vi "projet_licence_1.vi"() -> ()   [LabVIEW 2021]
uses:
  <vilib>/addons/control/pid/pid.llb/PID (DBL).vi
  <vilib>/addons/control/pid/NI_PID_pid.lvlib
panel:
  in  "Température\nde consigne":dbl=20.0 min=20.0 max=50.0 format="%#_4g"
  out "PWM correspondant":u8
  in  "Pin":u8=1 caption="Pin [0 - 11]" max=11
  out "Waveform Chart 2":dynamicdata(graph)
  in  "Commande onglet":T1(tab)
  out "Température mesurée":dbl
  out "Température mesurée":dbl(slide) scale=0.0..100.0
  out "Température actuelle":dbl
  out "Température mesurée":dbl(slide) scale=0.0..100.0
  in  "Température\nde consigne":dbl=20.0 min=20.0 max=50.0 format="%#_4g"
  out "Tension de consigne correspondante":dbl
  out "Température mesurée":dbl(slide) scale=0.0..100.0
  in  "Température de consigne":dbl(slide) scale=0.0..100.0
  out "Erreur":dbl
  out "Température":dbl(slide) scale=0.0..100.0
  out "Température actuelle":dbl
  in  "PID gains":T2={"derivative time (Td, min)"=0.0, "integral time (Ti, min)"=0.01, "proportional gain (Kc)"=1.0} {"proportional gain (Kc)" format="%.3f"; "integral time (Ti, min)" format="%.3f"; "derivative time (Td, min)" format="%.3f"}
  in  "stop":bool
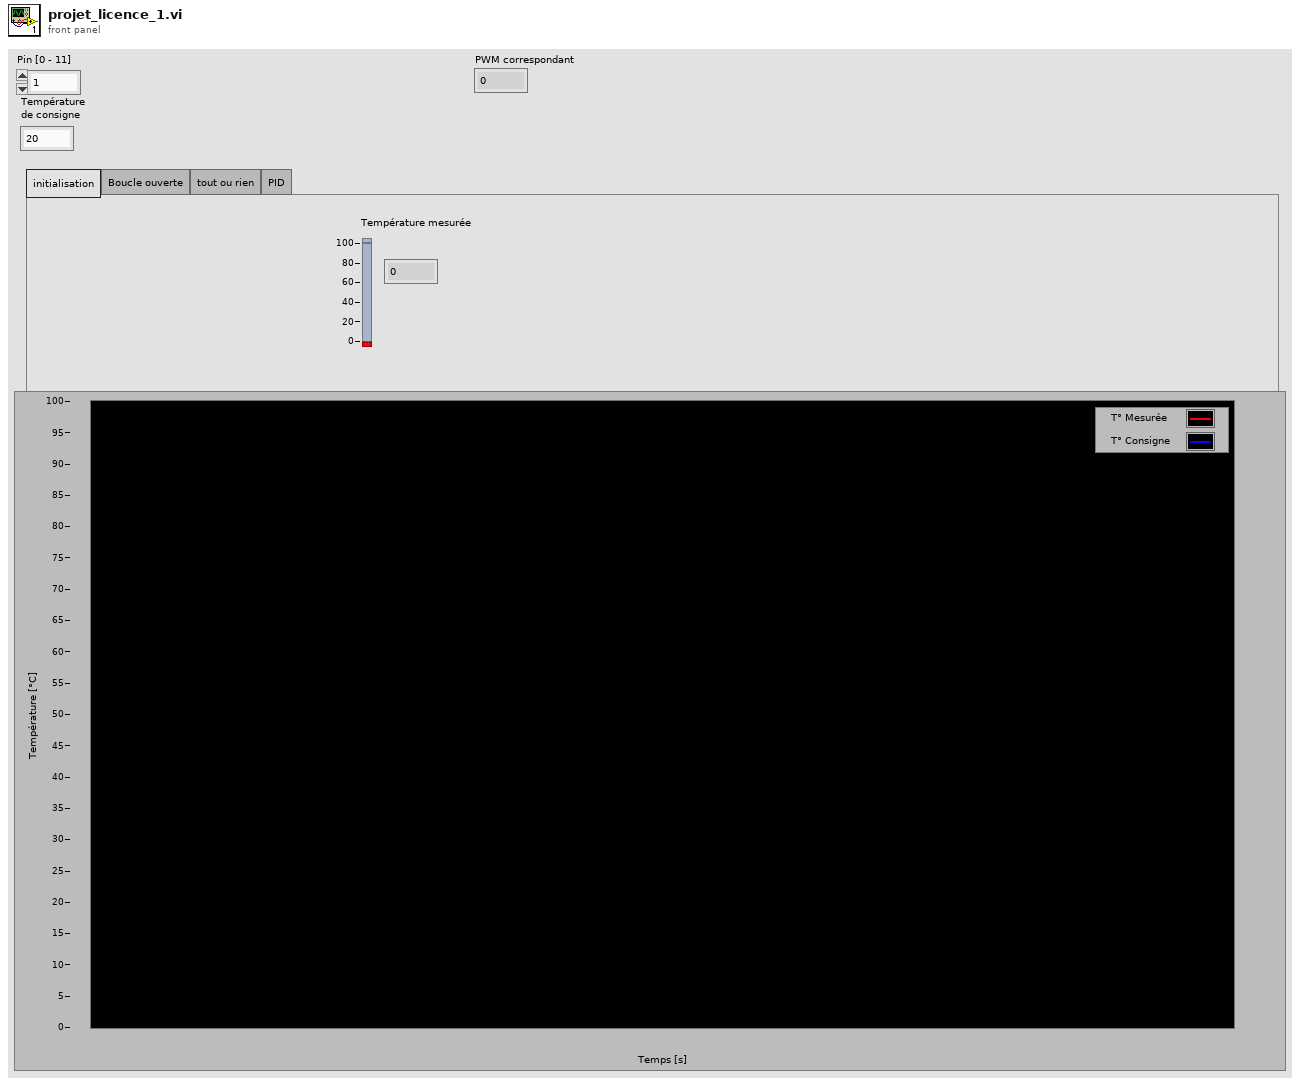
[diagram p1: front panel]
types:
  T1 = enum32{"initialisation", "Boucle ouverte", "tout ou rien", "PID"}
  T2 = cluster{"derivative time (Td, min)":dbl, "integral time (Ti, min)":dbl, "proportional gain (Kc)":dbl}
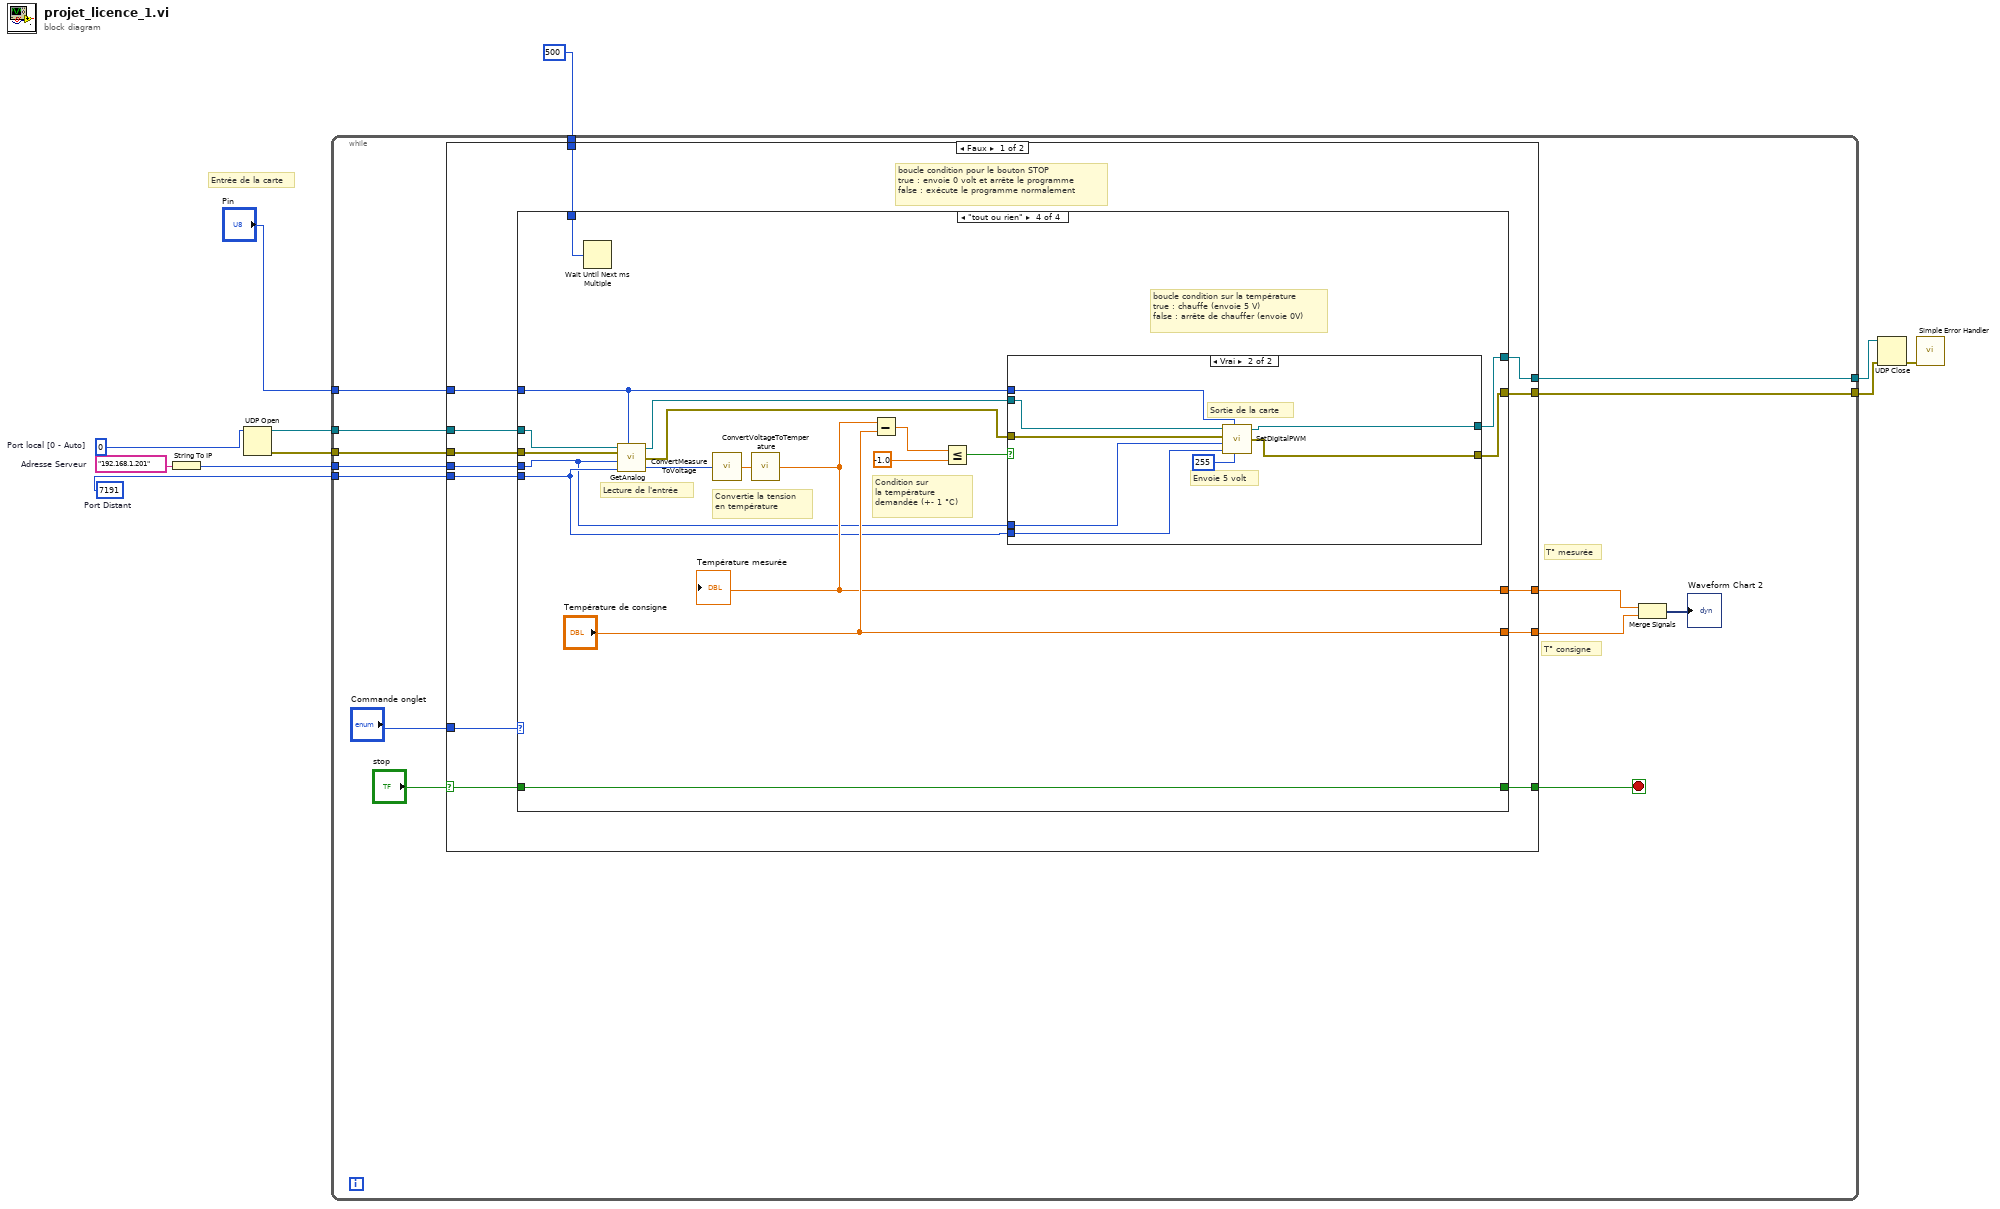
[diagram p0: block diagram]
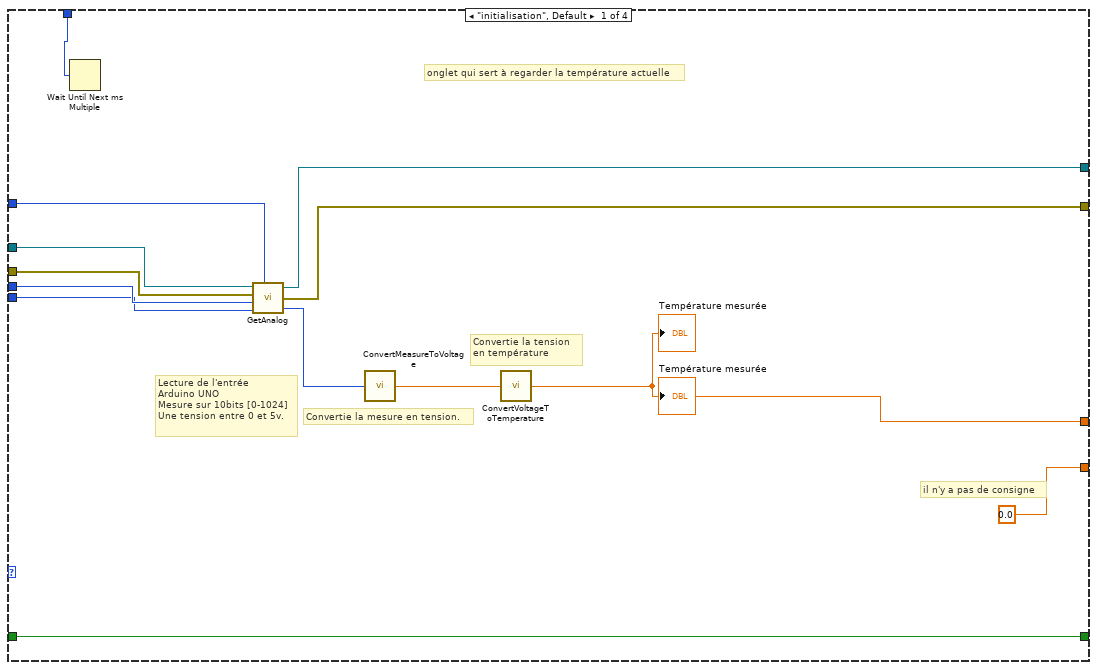
[diagram p2: hidden frame]
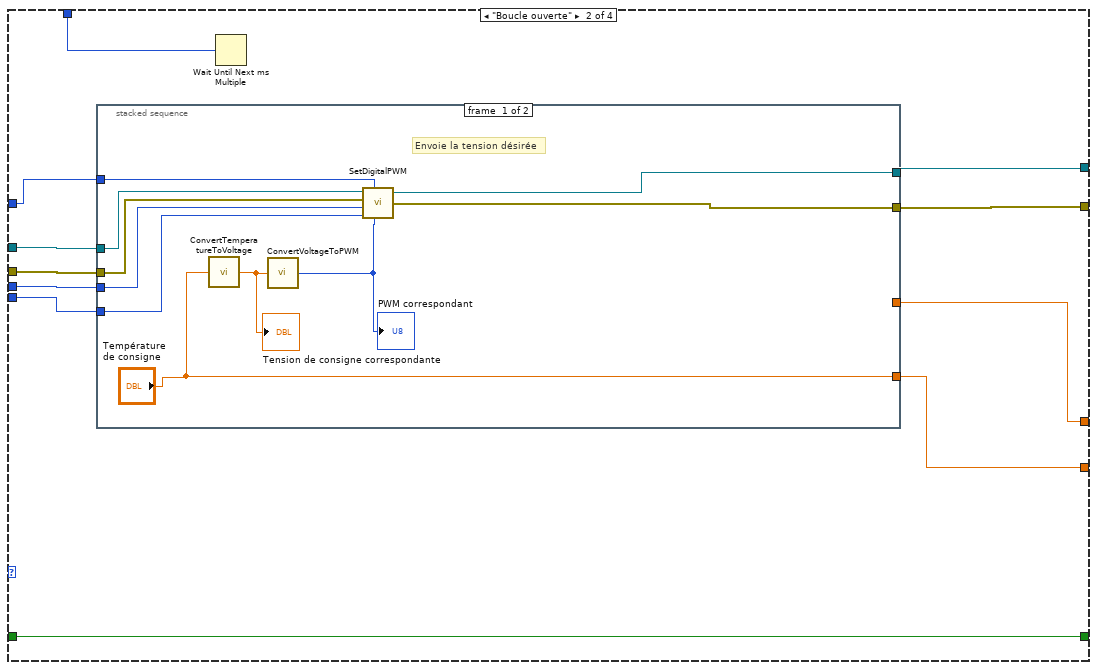
[diagram p3: hidden frame]
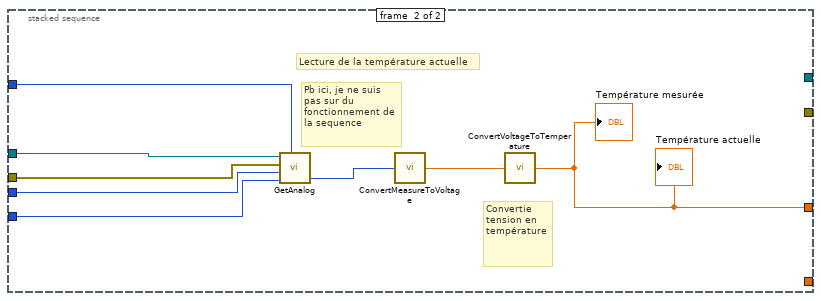
[diagram p4: hidden frame]
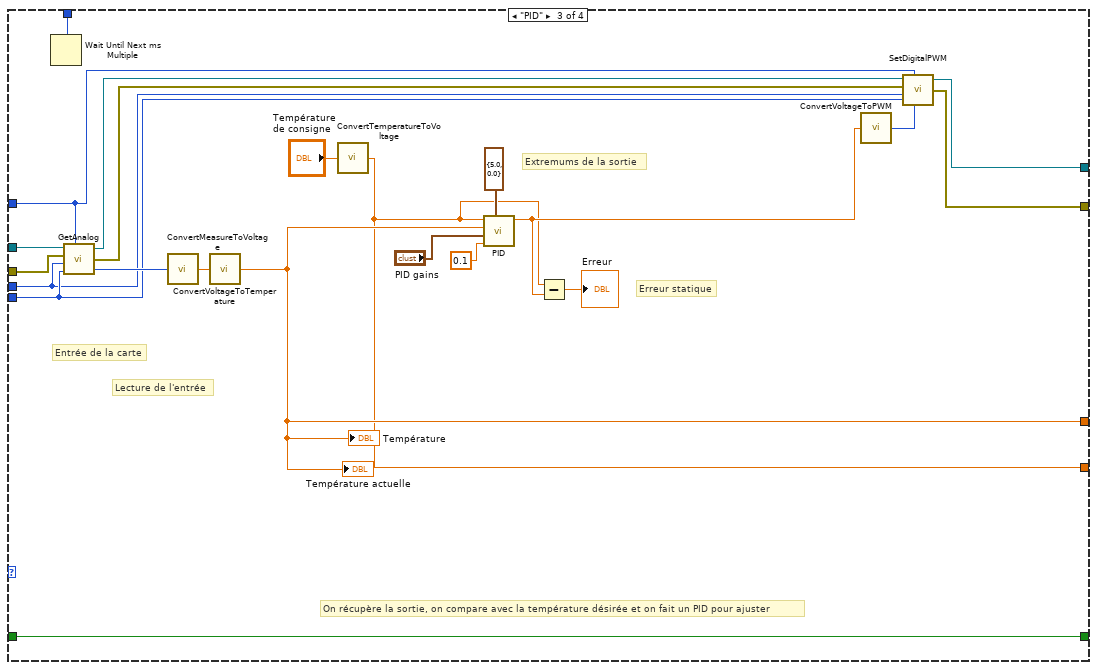
[diagram p5: hidden frame]
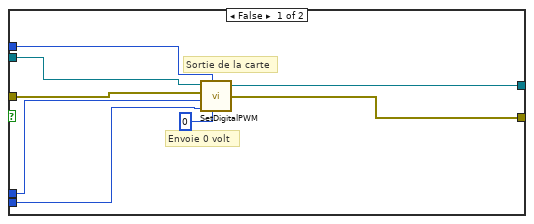
[diagram p6: hidden frame]
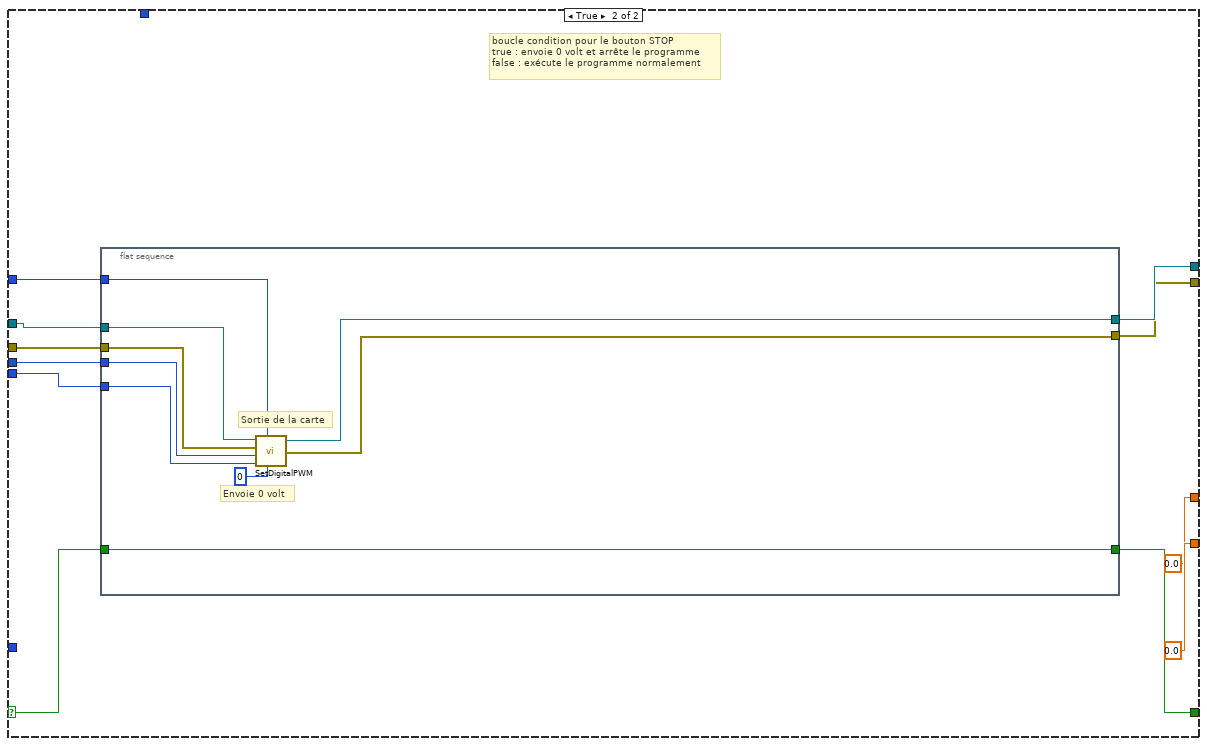
[diagram p7: hidden frame]
diagram:
  w6 = u16 7191  # Port Distant
  w10 = u16 0  # Port local [0 - Auto]
  w11 = "192.168.1.201"  # Adresse Serveur
  # "Entrée de la carte"
  n1 = String To IP(1:w11) -> (0:w7:u32)
  n2 = UDP Open(11:w10) -> (port=w9:refnum<k16>, 0:w8:errorcluster)  [unwired: 4 in, 1 out]
  n3 = while {
    tunnel: w9 -> [w20]
    tunnel: w8 -> [w19]
    tunnel: w7 -> [w18]
    tunnel: w6 -> [w17]
    tunnel: "Pin" -> [w15]
    tunnel: [w14] -> w1
    tunnel: [w13] -> w3
    tunnel: u32 500 ("millisecond multiple") -> [w12]
    stop <- w21 stop-if-true
    # "T° consigne"
    # "T° mesurée"
    n4 = case shown="Faux" "stop" {
      selector: "stop" -> [w35 w147]
      tunnel: "Commande onglet" -> [w38 _]
      tunnel: [w37 0.0 ("data")] -> w24
      tunnel: [w36 0.0 ("Température désirée")] -> w23
      tunnel: [w34 w146] -> w21
      tunnel: w20 -> [w33 w143]
      tunnel: w19 -> [w32 w142]
      tunnel: w18 -> [w31 w141]
      tunnel: w17 -> [w30 w140]
      tunnel: w15 -> [w29 w139]
      tunnel: [w28 w138] -> w14
      tunnel: [w27 w137] -> w13
      tunnel: w12 -> [w26 _]
      frame False {
        # "boucle condition pour le bouton STOP \ntrue : envoie 0 volt et arrête le programme\nfalse : exécute le programme normalement"
        n5 = case shown="\"tout ou rien\"" w38 {
          tunnel: [w39 w62 w89 w112] -> w37
          tunnel: [0.0 ("température désirée") w54 w81 "Température de consigne"] -> w36
          tunnel: w35 -> [w50 w61 w98 w116]
          tunnel: [w50 w61 w98 w116] -> w34
          tunnel: w33 -> [w49 w59 w93 w110]
          tunnel: w32 -> [w48 w58 w90 w109]
          tunnel: w31 -> [w47 w57 w84 w107]
          tunnel: w30 -> [w46 w56 w87 w108]
          tunnel: w29 -> [w44 w53 w92 w111]
          tunnel: [w42 w52 w86 w106] -> w28
          tunnel: [w43 w55 w85 w105] -> w27
          tunnel: w26 -> [w41 w60 w97 w115]
          frame "initialisation", Default {
            # "Convertie la mesure en tension."
            # "il n'y a pas de consigne"
            # "onglet qui sert à regarder la température actuelle"
            # "Convertie la tension \nen température"
            # "Lecture de l'entrée\nArduino UNO \nMesure sur 10bits [0-1024]\nUne tension entre 0 et 5v."
            n6 = Wait Until Next ms Multiple(millisecond multiple=w41) -> ()  [unwired: 1 out]
            n7 = call "GetAnalog.vi"("Connexion réseau UDP en entrée"=w49, "Pin"=w44, "entrée d'erreur (pas d'erreur)"=w48, "Adresse IP"=w47, "Port Distant"=w46) -> ("Connexion réseau UDP en sortie"=w42:refnum<k16>, "sortie d'erreur"=w43:errorcluster, "Return Value"=w45:u16)  [unwired: 1 in]
            n8 = call "ConvertMeasureToVoltage.vi"("Input Measure"=w45) -> ("Voltage"=w40:dbl)
            n9 = call "ConvertVoltageToTemperature.vi"("Voltage"=w40) -> ("Numérique"=w39:dbl)
            "Température mesurée" <- w39
            "Température mesurée" <- w39
          }
          frame "Boucle ouverte" {
            n10 = stacked-sequence {
              tunnel: [_ w80] -> w62
              tunnel: w59 -> [w72 w78]
              tunnel: w58 -> [w71 w77]
              tunnel: w57 -> [w70 w76]
              tunnel: w56 -> [w69 w75]
              tunnel: [w68 _] -> w52
              tunnel: [w67 _] -> w55
              tunnel: ["Température\nde consigne" _] -> w54
              tunnel: w53 -> [w66 w74]
              frame #0 {
                # "Envoie la tension désirée"
                n11 = call "ConvertTemperatureToVoltage.vi"("Température\nde consigne"="Température\nde consigne") -> ("Numérique"=w63:dbl)
                "Tension de consigne correspondante" <- w63
                n12 = call "ConvertVoltageToPWM.vi"("Numérique en entrée"=w63) -> ("Numérique en sortie"=w64:u8)
                "PWM correspondant" <- w64
                n13 = call "SetDigitalPWM.vi"("Connexion réseau UDP en entrée"=w72, "Pin"=w66, "entrée d'erreur (pas d'erreur)"=w71, "Adresse IP"=w70, "Value In"=w64, "Port Distant"=w69) -> ("Connexion réseau UDP en sortie"=w68:refnum<k16>, "error out"=w67:errorcluster)  [unwired: 1 out]
              }
              frame #1 {
                # "Pb ici, je ne suis pas sur du fonctionnement de la sequence"
                # "Convertie tension en\ntempérature"
                # "Lecture de la température actuelle"
                n14 = call "GetAnalog.vi"("Connexion réseau UDP en entrée"=w78, "Pin"=w74, "entrée d'erreur (pas d'erreur)"=w77, "Adresse IP"=w76, "Port Distant"=w75) -> ("Return Value"=w73:u16)  [unwired: 1 in, 2 out]
                n15 = call "ConvertMeasureToVoltage.vi"("Input Measure"=w73) -> ("Voltage"=w79:dbl)
                n16 = call "ConvertVoltageToTemperature.vi"("Voltage"=w79) -> ("Numérique"=w80:dbl)
                "Température actuelle" <- w80
                "Température mesurée" <- w80
              }
            }
            n17 = Wait Until Next ms Multiple(millisecond multiple=w60) -> ()  [unwired: 1 out]
          }
          frame "PID" {
            # "Lecture de l'entrée"
            # "On récupère la sortie, on compare avec la température désirée et on fait un PID pour ajuster"
            # "Erreur statique"
            # "Extremums de la sortie"
            # "Entrée de la carte"
            n18 = Wait Until Next ms Multiple(millisecond multiple=w97) -> ()  [unwired: 1 out]
            n19 = call "GetAnalog.vi"("Connexion réseau UDP en entrée"=w93, "Pin"=w92, "entrée d'erreur (pas d'erreur)"=w90, "Adresse IP"=w84, "Port Distant"=w87) -> ("Connexion réseau UDP en sortie"=w91:refnum<k16>, "sortie d'erreur"=w88:errorcluster, "Return Value"=w95:u16)  [unwired: 1 in]
            n20 = call "ConvertMeasureToVoltage.vi"("Input Measure"=w95) -> ("Voltage"=w96:dbl)
            n21 = call "ConvertVoltageToTemperature.vi"("Voltage"=w96) -> ("Numérique"=w89:dbl)
            "Température actuelle" <- w89
            "Température" <- w89
            n22 = call "ConvertTemperatureToVoltage.vi"("Température\nde consigne"="Température\nde consigne") -> ("Numérique"=w81:dbl)
            n23 = call-poly <vilib>:"PID.vi"("output range"=cluster{"output high":dbl, "output low":dbl} {"output high"=5.0, "output low"=0.0}, "dt (s)"=0.1, "PID gains"="PID gains", "process variable"=w89, "setpoint"=w81) -> ("output"=w82:dbl)  [unwired: 5 in, 1 out]
            n24 = Subtract(x=w81, y=w82) -> (x-y=→"Erreur":dbl)
            n25 = call "ConvertVoltageToPWM.vi"("Numérique en entrée"=w82) -> ("Numérique en sortie"=w94:u8)
            n26 = call "SetDigitalPWM.vi"("Connexion réseau UDP en entrée"=w91, "Pin"=w92, "entrée d'erreur (pas d'erreur)"=w88, "Adresse IP"=w84, "Value In"=w94, "Port Distant"=w87) -> ("Connexion réseau UDP en sortie"=w86:refnum<k16>, "error out"=w85:errorcluster)  [unwired: 1 out]
          }
          frame "tout ou rien" {
            # "Condition sur \nla température \ndemandée (+- 1 °C)"
            # "boucle condition sur la température\ntrue : chauffe (envoie 5 V)\nfalse : arrête de chauffer (envoie 0V)"
            # "Convertie la tension\nen température"
            # "Lecture de l'entrée"
            n27 = Wait Until Next ms Multiple(millisecond multiple=w115) -> ()  [unwired: 1 out]
            n28 = call "GetAnalog.vi"("Connexion réseau UDP en entrée"=w110, "Pin"=w111, "entrée d'erreur (pas d'erreur)"=w109, "Adresse IP"=w107, "Port Distant"=w108) -> ("Connexion réseau UDP en sortie"=w104:refnum<k16>, "sortie d'erreur"=w103:errorcluster, "Return Value"=w113:u16)  [unwired: 1 in]
            n29 = call "ConvertMeasureToVoltage.vi"("Input Measure"=w113) -> ("Voltage"=w114:dbl)
            n30 = call "ConvertVoltageToTemperature.vi"("Voltage"=w114) -> ("Numérique"=w112:dbl)
            "Température mesurée" <- w112
            n31 = Subtract(x=w112, y="Température de consigne") -> (x-y=w120:dbl)
            n32 = Less Or Equal?(x=w120, y=-1.0) -> (x <= y?=w118:bool)
            n33 = case shown="Vrai" w118 {
              tunnel: w111 -> [w127 w134]
              tunnel: w104 -> [w126 w135]
              tunnel: w103 -> [w125 w133]
              tunnel: w107 -> [w124 w132]
              tunnel: w108 -> [w123 w131]
              tunnel: [w122 w130] -> w106
              tunnel: [w121 w129] -> w105
              frame False {
                # "Envoie 0 volt"
                # "Sortie de la carte"
                n34 = call "SetDigitalPWM.vi"("Connexion réseau UDP en entrée"=w126, "Pin"=w127, "entrée d'erreur (pas d'erreur)"=w125, "Adresse IP"=w124, "Value In"=u8 0, "Port Distant"=w123) -> ("Connexion réseau UDP en sortie"=w122:refnum<k16>, "error out"=w121:errorcluster)  [unwired: 1 out]
              }
              frame True {
                # "Envoie 5 volt"
                # "Sortie de la carte"
                n35 = call "SetDigitalPWM.vi"("Connexion réseau UDP en entrée"=w135, "Pin"=w134, "entrée d'erreur (pas d'erreur)"=w133, "Adresse IP"=w132, "Value In"=u8 255, "Port Distant"=w131) -> ("Connexion réseau UDP en sortie"=w130:refnum<k16>, "error out"=w129:errorcluster)  [unwired: 1 out]
              }
            }
          }
        }
      }
      frame True {
        # "boucle condition pour le bouton STOP \ntrue : envoie 0 volt et arrête le programme\nfalse : exécute le programme normalement"
        n36 = flat-sequence {
          tunnel: w147 -> [w156]
          tunnel: [w156] -> w146
          tunnel: w143 -> [w155]
          tunnel: w142 -> [w154]
          tunnel: w141 -> [w153]
          tunnel: w140 -> [w152]
          tunnel: w139 -> [w151]
          tunnel: [w148] -> w138
          tunnel: [w149] -> w137
          frame #0 {
            # "Envoie 0 volt"
            # "Sortie de la carte"
            n37 = call "SetDigitalPWM.vi"("Connexion réseau UDP en entrée"=w155, "Pin"=w151, "entrée d'erreur (pas d'erreur)"=w154, "Adresse IP"=w153, "Value In"=u8 0, "Port Distant"=w152) -> ("Connexion réseau UDP en sortie"=w148:refnum<k16>, "error out"=w149:errorcluster)  [unwired: 1 out]
          }
        }
      }
    }
    n38 = Merge Signals(w24, w23) -> (→"Waveform Chart 2":dynamicdata)
  }
  n39 = UDP Close(connection ID=w1, 8:w3) -> (error out=w4:errorcluster)  [unwired: 1 out]
  n40 = call <vilib>:"Simple Error Handler.vi"("error in (no error)"=w4) -> ()  [unwired: 4 in, 5 out]
